vi "add data multiline.vi"(10 "data":dbl[][](array[numeric]), 11 "path":string[](array[string])) -> (0 "error out":errorcluster)   [LabVIEW 2014]
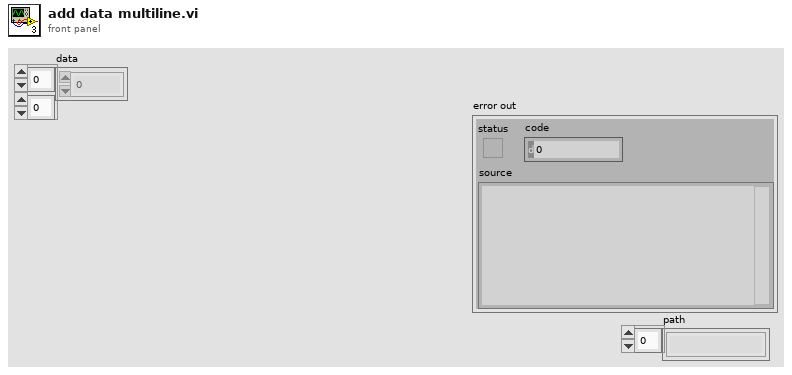
[diagram p1: front panel]
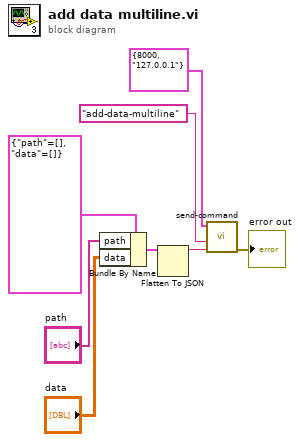
[diagram p0: block diagram]
diagram:
  n1 = Bundle By Name(cluster=cluster{"path":string[], "data":dbl[][]} {"path"=[], "data"=[]}, "path"="path", "data"="data") -> (w2:cluster{"path":string[], "data":dbl[][]})
  n2 = Flatten To JSON(anything=w2) -> (JSON string=w5:string)  [unwired: 2 in, 1 out]
  n3 = call "send-command.vi"("parameters"=w5, "command"="add-data-multiline", "target"=cluster{"port":i32, "host":string} {"port"=8000, "host"="127.0.0.1"}) -> ("error out"=→"error out":errorcluster)  [unwired: 7 in, 1 out]
